vi "MTM2_logEvent_detailedState.vi"(8 "error in (no error)":errorcluster, 11 "logevent_detailedState_Ctl":T1) -> (0 "error out":errorcluster, 2 "function return":i32, 3 "logevent_detailedState_Ctl out":T1)   [LabVIEW 2018, in "SALLV_MTM2.lvlib"]
doc: "int MTM2_shm_logEvent_detailedStateLV(MTM2_logevent_detailedStateLV *logevent_detailedState_Ctl );"
uses:
  DataTypes/logevent_detailedState.ctl
  SALLV_MTM2.lvlib
  SALLV_MTM2.so
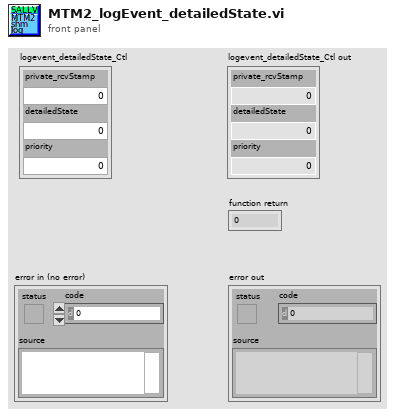
[diagram p1: front panel]
types:
  T1 = typedef "SALLV_MTM2.lvlib/logevent_detailedState.ctl" = cluster{"private_rcvStamp":dbl, "detailedState":i32, "priority":i32}
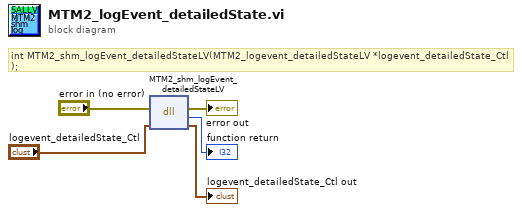
[diagram p0: block diagram]
diagram:
  # "int MTM2_shm_logEvent_detailedStateLV(MTM2_logevent_detailedStateLV *logevent_detailedState_Ctl );"
  n1 = dll-call lib="home/ttsai/Documents/salLabviewApi/SALLV_MTM2/SALLV_MTM2.*" fn="MTM2_shm_logEvent_detailedStateLV"(error in="error in (no error)", "logevent_detailedState_Ctl"="logevent_detailedState_Ctl") -> (error out=→"error out":errorcluster, →"function return":i32, "logevent_detailedState_Ctl"=→"logevent_detailedState_Ctl out":T1)  [unwired: 2 in, 1 out]
